vi "split_images.vi"() -> ()   [LabVIEW 2024]
uses:
  <vilib>/vision/NI_Vision_Development_Module.lvlib
panel:
  out "Original Image":T1(plugin-control)
  out "Output Image":T1(plugin-control)
  in  "Overlap %":dbl
  in  "Split into:":u32
  in  "Image/ File Directory":path
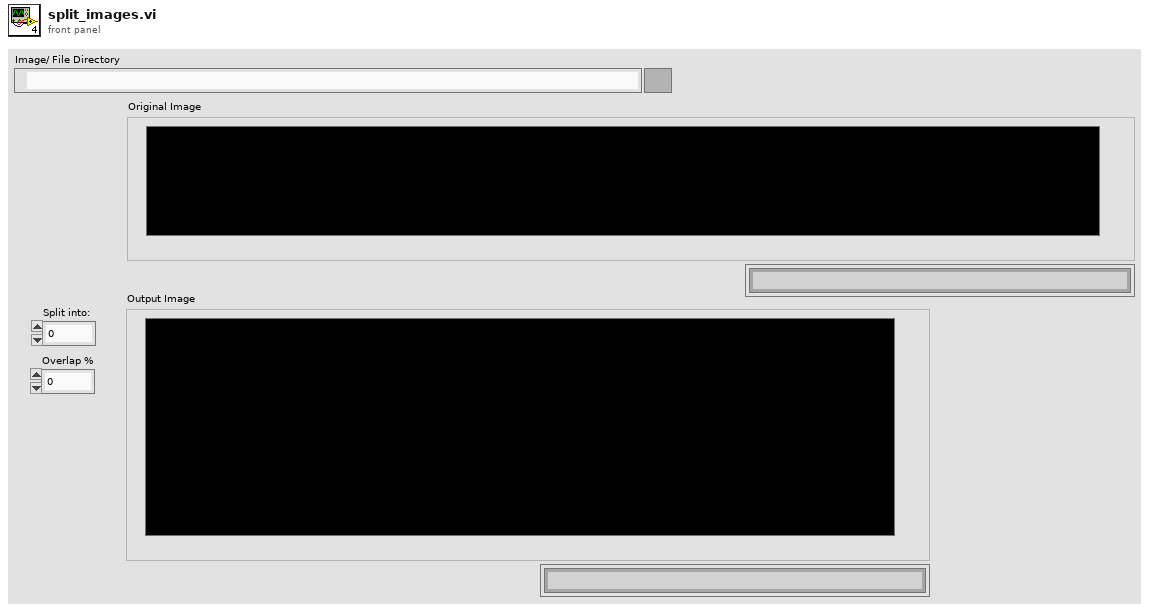
[diagram p1: front panel]
types:
  T1 = typedef "IMAQ Image.ctl" = refnum<image>
  T2 = cluster{"Brightness":sgl, "Contrast":sgl, "Gamma":sgl}
  T3 = typedef "Image Type" = u32
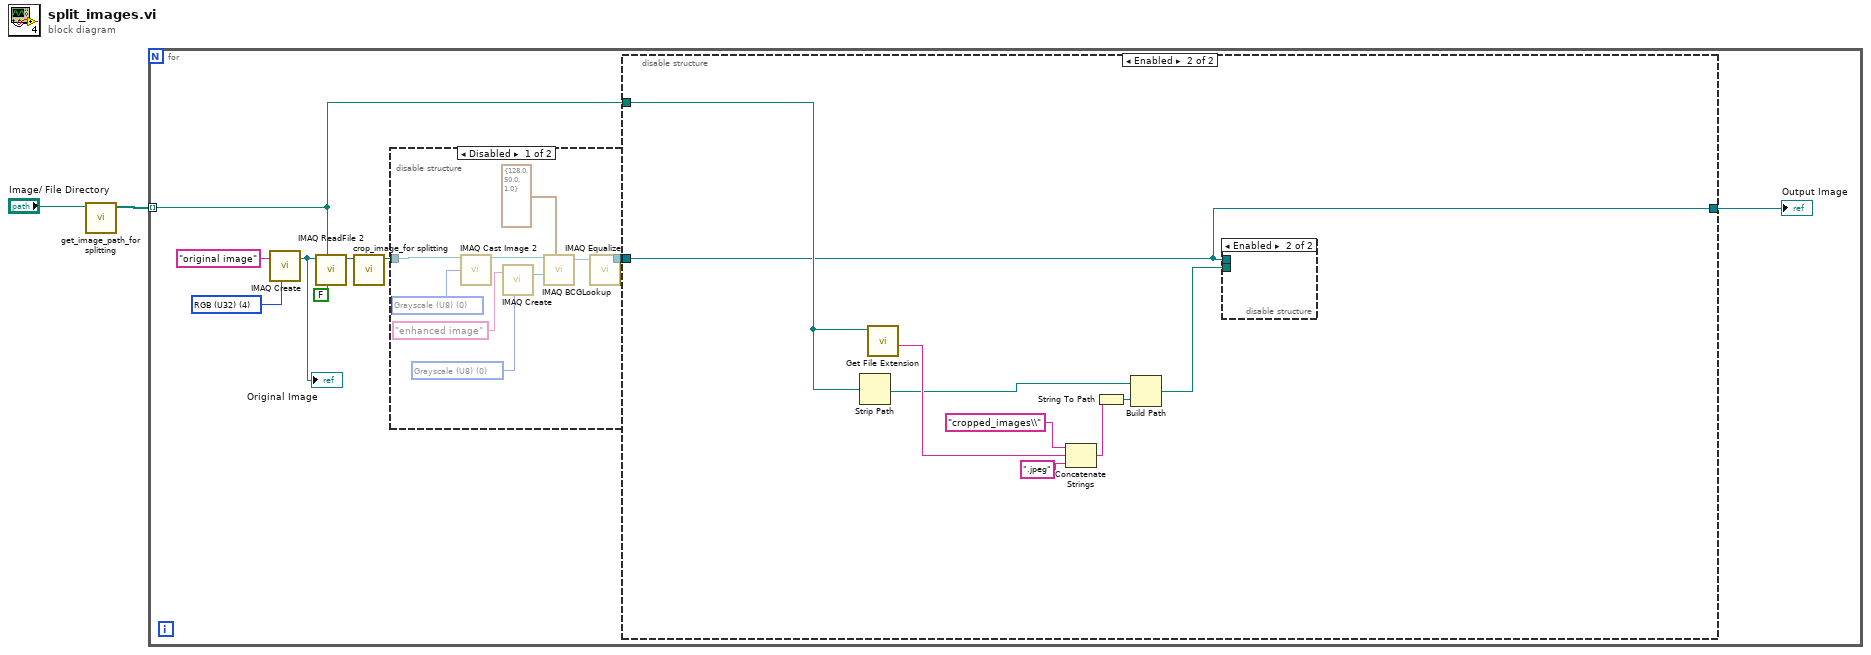
[diagram p0: block diagram]
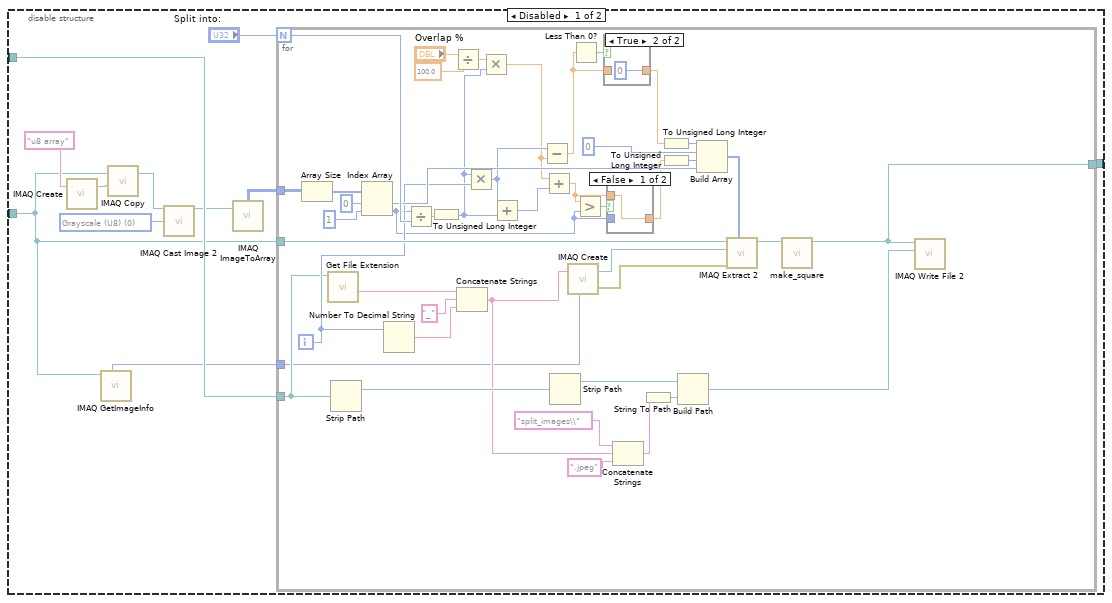
[diagram p3: hidden frame]
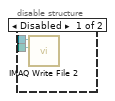
[diagram p6: hidden frame]
diagram:
  n1 = call "get_image_path_for splitting.vi"("Image/ File Directory"="Image/ File Directory") -> ("Array"=w1:path[])  [unwired: 10 in]
  n2 = for {
    tunnel: w1 -> [w7] mode=indexing
    w10 = T3 4 items=["Grayscale (U8)", "Grayscale (I16)", "Grayscale (SGL)", "Complex (CSG)", "RGB (U32)", "HSL (U32)", "RGB (U64)", "Grayscale (U16)"] ("Image Type")
    n3 = call "IMAQ Create"("Image Name"="original image", "Image Type"=w10) -> ("New Image"=w5:T1)  [unwired: 3 in, 1 out]
    "Original Image" <- w5
    n4 = call "IMAQ ReadFile 2"("Use File Path Image Type"=FALSE, "File Path"=w7, "Image"=w5) -> ("Image Out"=w8:T1)  [unwired: 4 in, 4 out]
    n5 = call "crop_image_for splitting.vi"("Image in"=w8) -> ("Image out"=w3:T1)  [unwired: 10 in]
    n6 = disable-structure shown="Disabled" {
      disable-tunnel: [w16 w21] -> w6
      disable-tunnel: w3 -> [w14 w21]
      frame Disabled {
        w12 = T3 0 items=["Grayscale (U8)", "Grayscale (I16)", "Grayscale (SGL)", "Complex (CSG)", "RGB (U32)", "HSL (U32)", "RGB (U64)", "Grayscale (U16)"] ("Image Type")
        w15 = T3 0 items=["Grayscale (U8)", "Grayscale (I16)", "Grayscale (SGL)", "Complex (CSG)", "RGB (U32)", "HSL (U32)", "RGB (U64)", "Grayscale (U16)"] ("Image Type")
        n7 = call "IMAQ Cast Image 2"("Image Src"=w14, "Image Type"=w12) -> ("Image Dst Out"=w13:T1)  [unwired: 12 in, 1 out]
        n8 = call "IMAQ Create"("Image Name"="enhanced image", "Image Type"=w15) -> ("New Image"=w18:T1)  [unwired: 3 in, 1 out]
        n9 = call "IMAQ BCGLookup"("Image Src"=w13, "BCG Values"=T2 {"Brightness"=128.0, "Contrast"=50.0, "Gamma"=1.0}, "Image Dst"=w18) -> ("Image Dst Out"=w17:T1)  [unwired: 4 in, 1 out]
        n10 = call "IMAQ Equalize"("Image Src"=w17) -> ("Image Dst Out"=w16:T1)  [unwired: 9 in, 1 out]
      }
      frame Enabled {
      }
    }
    n11 = disable-structure shown="Enabled" {
      disable-tunnel: w7 -> [w31 w85]
      disable-tunnel: w6 -> [w23 w81]
      disable-tunnel: [w29 w81] -> w4
      frame Disabled {
        w27 = T3 0 items=["Grayscale (U8)", "Grayscale (I16)", "Grayscale (SGL)", "Complex (CSG)", "RGB (U32)", "HSL (U32)", "RGB (U64)", "Grayscale (U16)"] ("Image Type")
        n12 = call "IMAQ Create"("Image Name"="u8 array") -> ("New Image"=w28:T1)  [unwired: 4 in, 1 out]
        n13 = call "IMAQ GetImageInfo"("Image"=w23) -> ("Image Type"=w22:T3)  [unwired: 3 in, 7 out]
        n14 = call "IMAQ Copy"("Image Dst"=w28, "Image Src"=w23) -> ("Image Dst Out"=w26:T1)  [unwired: 4 in, 1 out]
        n15 = call "IMAQ Cast Image 2"("Image Src"=w26, "Image Type"=w27) -> ("Image Dst Out"=w25:T1)  [unwired: 12 in, 1 out]
        n16 = call "IMAQ ImageToArray"("Image"=w25) -> ("Image Pixels (U8)"=w30:u8[][])  [unwired: 3 in, 4 out]
        n17 = for {
          N: "Split into:" -> [w68]
          tunnel: w31 -> [w61]
          tunnel: w30 -> [w73]
          tunnel: w23 -> [w69]
          tunnel: [w34] -> w29
          tunnel: w22 -> [w33]
          i -> [w63]
          n18 = Array Size(array=w73) -> (size(s)=w72:i32[])
          n19 = call <vilib>:"Get File Extension.vi"("file"=w61) -> ("filename without extension"=w60:string)  [unwired: 6 in, 4 out]
          n20 = Strip Path(path=w61) -> (stripped path=w62:path)  [unwired: 1 out]
          n21 = Index Array(array=w72, index #1=0 ("index"), index #2=1 ("index")) -> (element #1=w65:i32, element #2=w42:i32)
          n22 = Number To Decimal String(number=w63) -> (decimal integer string=w74:string)  [unwired: 1 in]
          n23 = Divide(x=w42, y=w68) -> (x/y=w64:dbl)
          n24 = To Unsigned Long Integer(number=w64) -> (unsigned 32bit integer=w49:u32)
          n25 = Divide(x="Overlap %", y=100.0) -> (x/y=w50:dbl)
          n26 = Concatenate Strings(w60, "_", w74) -> (w59:string)
          n27 = Multiply(x=w49, y=w63) -> (x*y=w48:u32)
          n28 = Multiply(x=w50, y=w49) -> (x*y=w40:dbl)
          n29 = Add(x=w48, y=w49) -> (x+y=w47:u32)
          n30 = Subtract(x=w48, y=w40) -> (x-y=w45:dbl)
          n31 = Add(x=w40, y=w47) -> (x+y=w41:dbl)
          n32 = Strip Path(path=w62) -> (stripped path=w56:path)  [unwired: 1 out]
          n33 = call "IMAQ Create"("Image Name"=w59, "Image Type"=w33) -> ("New Image"=w76:T1, "error out"=w67:errorcluster)  [unwired: 3 in]
          n34 = Less Than 0?(x=w45) -> (x < 0?=w44:bool)
          n35 = Greater?(x=w41, y=w42) -> (0:w43:bool)
          n36 = case shown="True" w44 {
            tunnel: [w79 u32 0 ("element")] -> w38
            tunnel: w45 -> [w79 _]
            frame False {
            }
            frame True {
            }
          }
          n37 = case shown="False" w43 {
            tunnel: [w77 w78] -> w36
            tunnel: w42 -> [_ w78]
            tunnel: w41 -> [w77 _]
            frame False {
            }
            frame True {
            }
          }
          n38 = Concatenate Strings("split_images\\" ("string"), w59, ".jpeg" ("string")) -> (w55:string)
          n39 = String To Path(string=w55) -> (path=w54:path)
          n40 = To Unsigned Long Integer(number=w38) -> (unsigned 32bit integer=w39:u32)
          n41 = To Unsigned Long Integer(number=w36) -> (unsigned 32bit integer=w37:u32)
          n42 = Build Path(base path=w56, name or relative path=w54) -> (appended path=w53:path)
          n43 = Build Array(w39, u32 0 ("element"), w37, w65) -> (w46:u32[])
          n44 = call "IMAQ Extract 2"("Optional Rectangle"=w46, "error in (no error)"=w67, "Image Dst"=w76, "Image Src"=w69) -> ("Image Dst Out"=w35:T1)  [unwired: 6 in, 1 out]
          n45 = call "make_square.vi"("Refnum in"=w35) -> ("Refnum out"=w34:T1)  [unwired: 10 in]
          n46 = call-poly "IMAQ Write File 2"("File Path"=w53, "Image"=w34) -> ()  [unwired: 8 in, 2 out]
        }
      }
      frame Enabled {
        n47 = Strip Path(path=w85) -> (stripped path=w82:path)  [unwired: 1 out]
        n48 = call <vilib>:"Get File Extension.vi"("file"=w85) -> ("filename without extension"=w84:string)  [unwired: 6 in, 4 out]
        n49 = Concatenate Strings("cropped_images\\" ("string"), w84, ".jpeg" ("string")) -> (w87:string)
        n50 = String To Path(string=w87) -> (path=w86:path)
        n51 = Build Path(base path=w82, name or relative path=w86) -> (appended path=w83:path)
        n52 = disable-structure shown="Enabled" {
          disable-tunnel: w83 -> [w91 _]
          disable-tunnel: w81 -> [w90 _]
          frame Disabled {
            n53 = call-poly "IMAQ Write File 2"("File Path"=w91, "Image"=w90) -> ()  [unwired: 8 in, 2 out]
          }
          frame Enabled {
          }
        }
      }
    }
    "Output Image" <- w4
  }
